vi "GET_STATUS_n.vi"(2 "execute":bool, 11 "error in (no error)":errorcluster) -> (4 "function return":string, 8 "uLPtr":u32[](array[numeric]), 10 "serial no":string, 15 "error out":errorcluster)   [LabVIEW 2017, in "ZBOX_IS.lvlib"]
uses:
  ZBOX_IS.lvlib
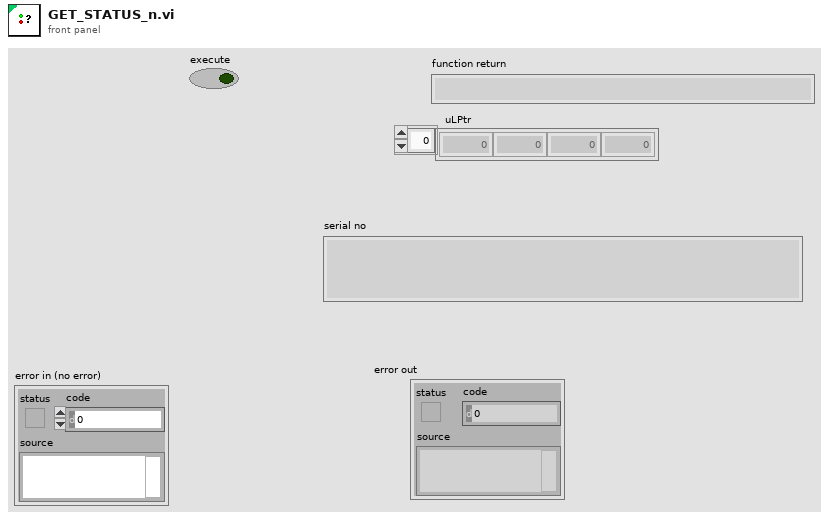
[diagram p1: front panel]
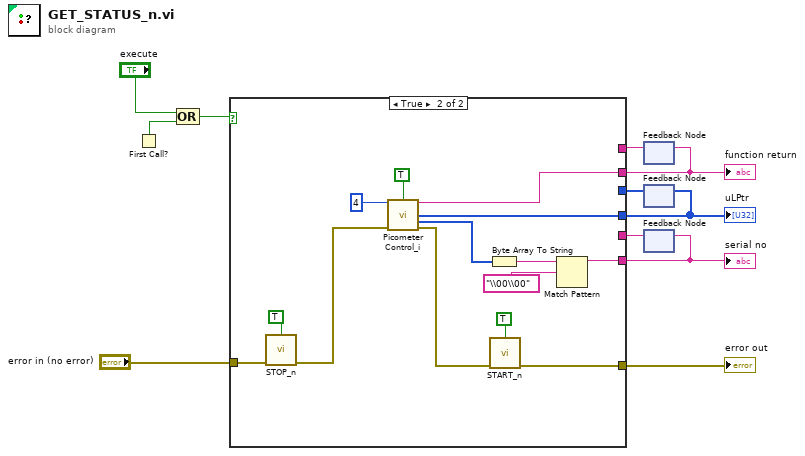
[diagram p0: block diagram]
diagram:
  n1 = First Call?() -> (First Call?: T/F=w1:bool)
  n2 = Compound Arithmetic op=OR("execute", w1) -> (w3:bool)
  n3 = feedback #1() -> (w6:string)  [unwired: 1 in]
  n4 = feedback #2() -> (w5:u32[])  [unwired: 1 in]
  n5 = feedback #3() -> (w4:string)  [unwired: 1 in]
  n6 = case shown="True" w3 {
    tunnel: [w15 w28] -> w10
    tunnel: [w14 w27] -> w7
    tunnel: [w13 w16] -> w8
    tunnel: "error in (no error)" -> [w12 w25]
    tunnel: [w12 w22] -> w9
    tunnel: w6 -> [w15 _]
    tunnel: w5 -> [w14 _]
    tunnel: w4 -> [w13 _]
    frame False {
    }
    frame True {
      n7 = call "STOP_n.vi"("execute"=TRUE, "error in (no error)"=w25) -> ("error out"=w24:errorcluster)  [unwired: 12 in, 1 out]
      n8 = call "Picometer Control_i.vi"("Cmd"=u8 4, "execute"=TRUE, "error in (no error)"=w24) -> ("function return"=w28:string, "uLPtr"=w27:u32[], "BytePtr"=w26:u8[], "error out"=w23:errorcluster)  [unwired: 8 in, 1 out]
      n9 = Byte Array To String(unsigned byte array=w26) -> (string=w18:string)
      n10 = call "START_n.vi"("execute"=TRUE, "error in (no error)"=w23) -> ("error out"=w22:errorcluster)  [unwired: 12 in, 1 out]
      n11 = Match Pattern(string=w18, regular expression="\\00\\00") -> (before substring=w16:string)  [unwired: 1 in, 3 out]
    }
  }
  "error out" <- w9
  "function return" <- w10
  "uLPtr" <- w7
  "serial no" <- w8
  n12 = feedback-in #1(w10) -> ()
  n13 = feedback-in #2(w7) -> ()
  n14 = feedback-in #3(w8) -> ()
